vi "FPGA_8a_2ws_BIdireccional_sinWheelsensor.vi"() -> ()   [LabVIEW 2015]
uses:
  <vilib>/LabVIEW Targets/FPGA/cRIO/shared/nicrio_ModuleControls/nicrio_cRIO-9234_DataRatesRing2.ctl
  <vilib>/LabVIEW Targets/FPGA/cRIO/shared/nicrio_ModuleControls/nicrio_BasicConversionTime.ctl
  <vilib>/rvi/Emulation/niFpgaGetClockAttributes.vi
  <vilib>/rvi/Emulation/niFpgaSctlEmulationGetInTimedLoop.vi
  <vilib>/rvi/Emulation/niFpgaEmulationReportErrorSimple.vi
  <vilib>/rvi/Emulation/niFpgaProcessEmulError.vi
  <vilib>/rvi/eio/common/nirviEmuTemplateMethod_errors.vi
  <vilib>/rvi/Emulation/niFpgaCriticalErrorInLSC.vi
  <vilib>/rvi/eio/common/nirviEmuTemplatePropertySet_errors.vi
  <vilib>/rvi/interface/RandomDataEmulation/niFpgaRandomDataHandleErrors.vi
  <vilib>/eio/EIONode/EIONode.xnode
  <vilib>/eio/EIOPropertyNode/EIOPropertyNode.xnode
  <vilib>/rvi/DataTransferAndStorage/Container/XNode/niFpgaContainer.xnode
  <vilib>/rvi/interface/RandomDataEmulation/nirviRandomDataFpgaReadWriteTemplate.vi
  <vilib>/rvi/eio/common/nirviEmuTemplatePropertyGet_errors.vi
  <vilib>/rvi/eio/common/nirviEmuTemplatePropertyGet_noerrors.vi
  <vilib>/rvi/eio/common/nirviEmuTemplatePropertySet_noerrors.vi
panel:
  out "RuedaDetectada2?":bool
  out "RuedaDetectada1?":bool
  out "Numeric 2":i32
  out "WhlCnt1":fxp<+/-,24,-4> format="%.27g"
  in  "Offset_WS1":fxp<+/-,24,-4>=0.000999998301267624 format="%.27g"
  out "Rueda1?":i16
  out "WhlCnt2":fxp<+/-,24,-4> format="%.27g"
  out "Rueda2?":i16
  out "Parar":bool
  out "Nº Ruedas 1":i32
  out "NºRuedas 2":i32
  in  "Offset_WS2":fxp<+/-,24,-4>=0.000999998301267624 format="%.27g"
  in  "Cycles to Filter":u16=5
  in  "Canal cero WS1?":bool=TRUE
  in  "Canal cero WS2?":bool=TRUE
  in  "Conversion Time":T1
  in  "Count(mSec)":u32=2
  in  "Stop":bool
  out "Buffer Underflow":bool
  in  "Digital?":bool=TRUE
  out "medidas":fxp<+/-,24,4>[](array[numeric])
  out "Buffer Overflow":bool
  out "Error Out":errorcluster
  in  "Data Rate":T2=2 items=["51.200 kS/s (NI 9234)"=1, "25.600 kS/s (NI 9234)"=2, "17.067 kS/s (NI 9234)"=3, "12.800 kS/s (NI 9234)"=4, "10.240 kS/s (NI 9234)"=5, "8.533 kS/s (NI 9234)"=6, "7.314 kS/s (NI 9234)"=7, "6.400 kS/s (NI 9234)"=8, "5.689 kS/s (NI 9234)"=9, "5.120 kS/s (NI 9234)"=10, "4.654 kS/s (NI 9234)"=11, "4.267 kS/s (NI 9234)"=12, "3.938 kS/s (NI 9234)"=13, "3.657 kS/s (NI 9234)"=14, "3.413 kS/s (NI 9234)"=15, "3.200 kS/s (NI 9234)"=16, "3.012 kS/s (NI 9234)"=17, "2.845 kS/s (NI 9234)"=18, "2.695 kS/s (NI 9234)"=19, "2.560 kS/s (NI 9234)"=20, "2.438 kS/s (NI 9234)"=21, "2.328 kS/s (NI 9234)"=22, "2.226 kS/s (NI 9234)"=23, "2.133 kS/s (NI 9234)"=24, "2.048 kS/s (NI 9234)"=25, "1.969 kS/s (NI 9234)"=26, "1.896 kS/s (NI 9234)"=27, "1.829 kS/s (NI 9234)"=28, "1.765 kS/s (NI 9234)"=29, "1.707 kS/s (NI 9234)"=30, "1.652 kS/s (NI 9234)"=31]
  out "DC OK":bool
  in  "Fotocélula":bool
  out "Detector de\npresencia":bool
  out "Chassis Temperature":i16
  out "Direccion 0?":bool
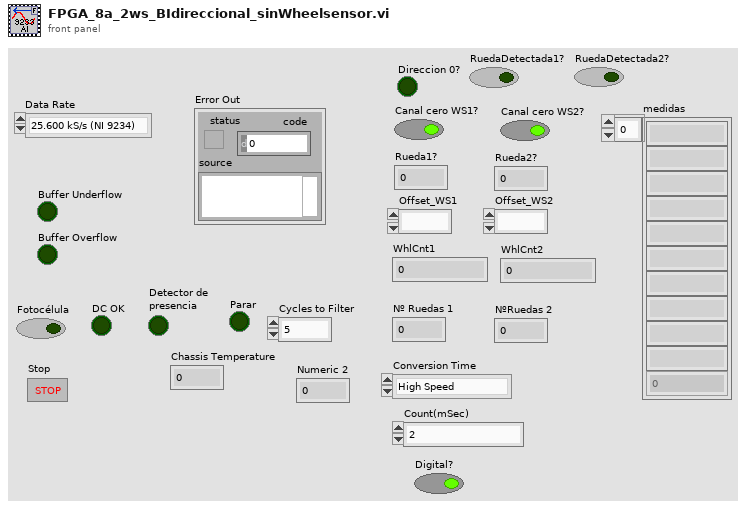
[diagram p1: front panel]
types:
  T1 = typedef "nicrio_BasicConversionTime.ctl" = enum8{"High Speed", "High Resolution"}
  T2 = typedef "nicrio_cRIO-9234_DataRatesRing2.ctl" = u8
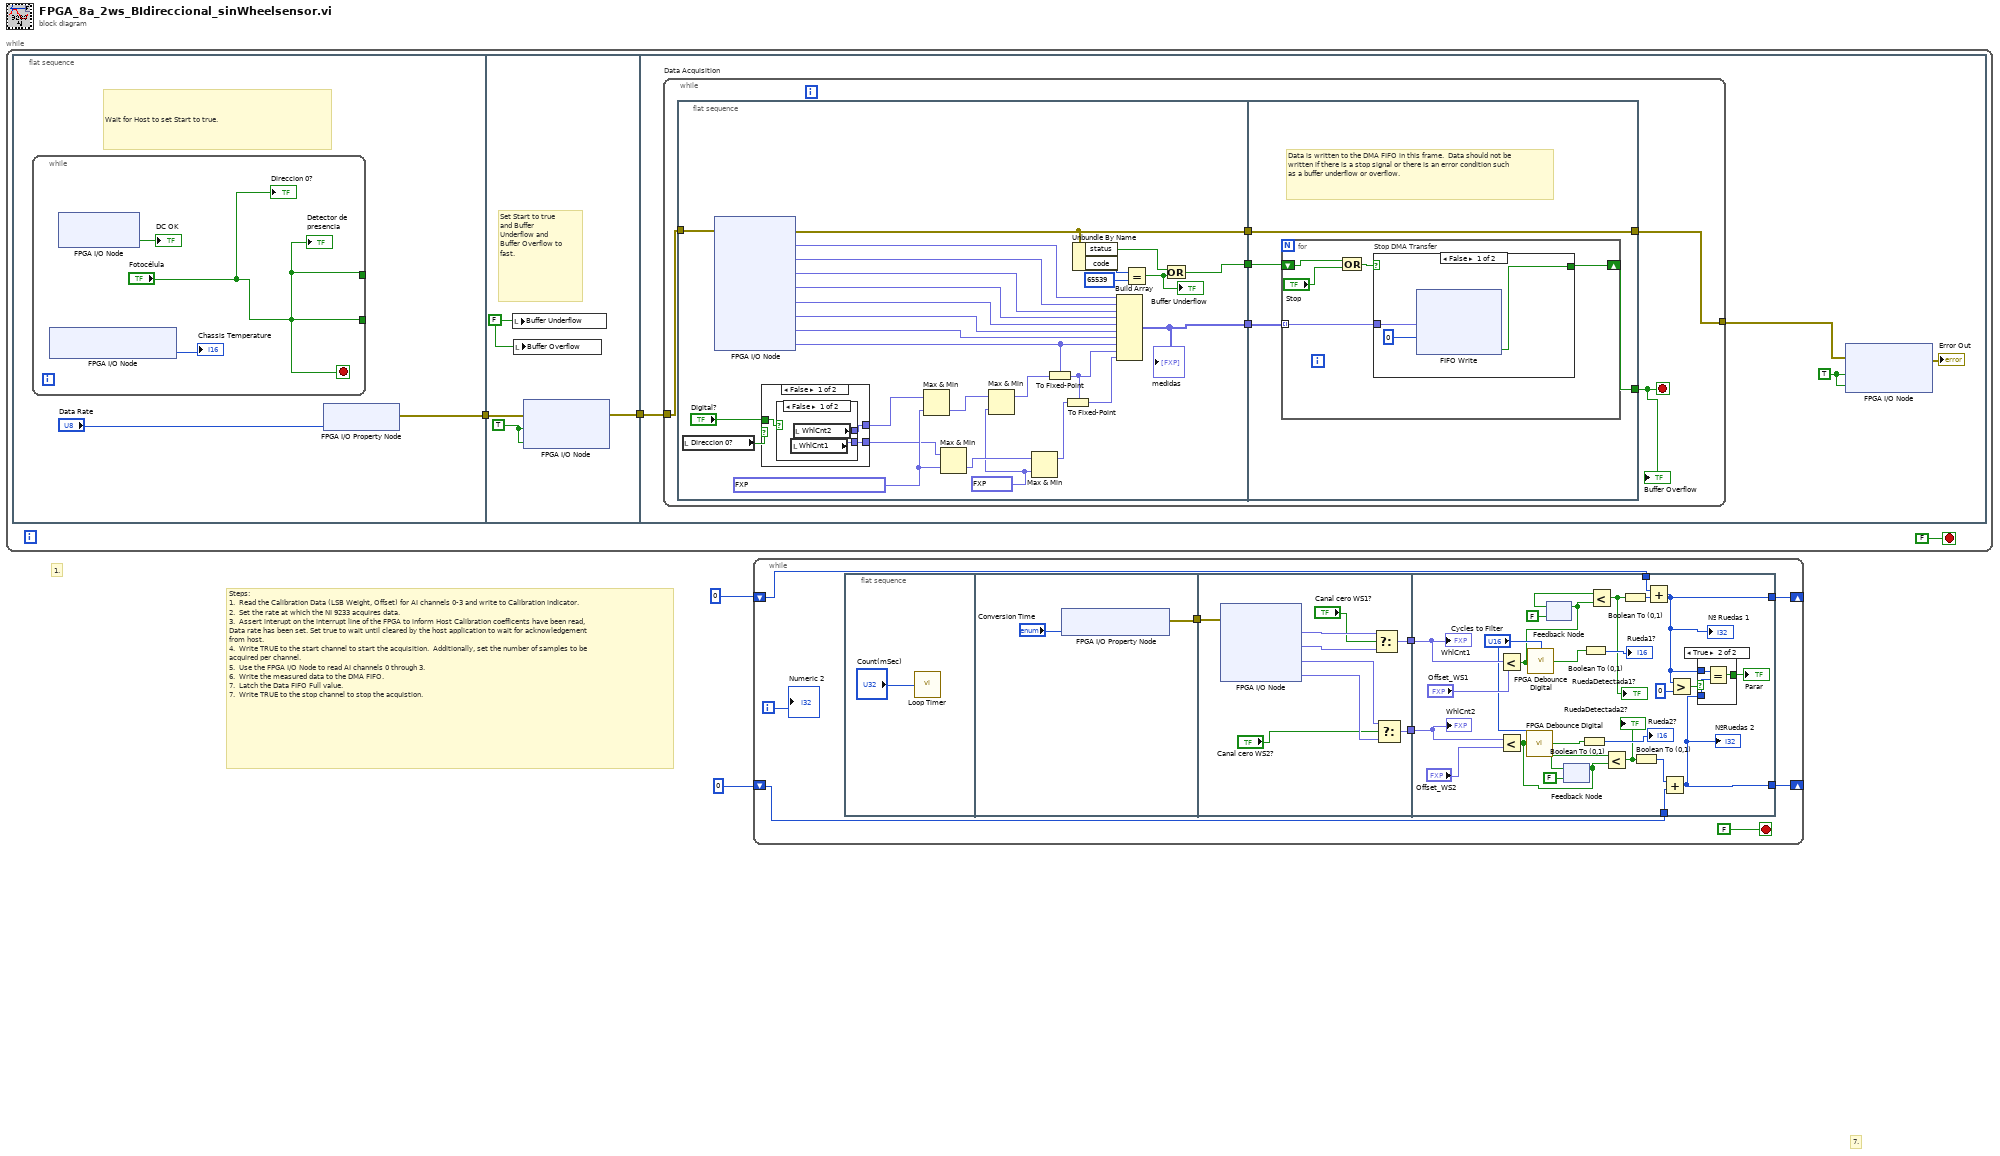
[diagram p0: block diagram]
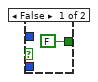
[diagram p2: hidden frame]
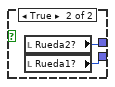
[diagram p3: hidden frame]
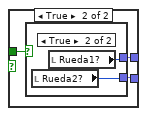
[diagram p4: hidden frame]
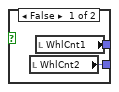
[diagram p5: hidden frame]
diagram:
  # "Steps: \n1.  Read the Calibration Data (LSB Weight, Offset) for AI channels 0-3 and write to Calibration indicator.\n2.  Set the rate at which the NI 9233 acquires data. \n3.  Assert interupt on the interrupt line of the FPGA to inform Host Calibration coefficents have been read, Data rate has been set. Set true to wait until cleared by the host application to wait for acknowledgement from host.\n4.  Write TRUE to the start channel to start the acquisition.  Additionally, set the number of samples to be acquired per channel.\n5.  Use the FPGA I/O Node to read AI channels 0 through 3. \n6.  Write the measured data to the DMA FIFO.\n7.  Latch the Data FIFO Full value.\n7.  Write TRUE to the stop channel to stop the acquistion."
  # "1."
  # "7."
  n1 = while {
    stop <- FALSE stop-if-true
    n2 = flat-sequence "MainSeq" {
      tunnel: [w7] -> w4
      tunnel: w4 -> [w13]
      tunnel: [w12] -> w3
      tunnel: w3 -> [w18]
      frame #0 {
        # "Wait for Host to set Start to true."
        n3 = while "initWait" {
          tunnel: ["Fotocélula"] -> _
          tunnel: ["Fotocélula"] -> _
          stop <- "Fotocélula" stop-if-true
          n4 = xnode "FPGA I/O Node"() -> ("Chassis Temperature"=→"Chassis Temperature":i16)  [unwired: 1 in, 1 out]
          n5 = xnode "FPGA I/O Node"() -> ("Mod3/DI2"=→"DC OK":bool)  [unwired: 2 in, 2 out]
          "Detector de\npresencia" <- "Fotocélula"
          "Direccion 0?" <- "Fotocélula"
        }
        n6 = xnode "FPGA I/O Property Node"("Data Rate"="Data Rate") -> ("error out"=w7:errorcluster)  [unwired: 2 in, 1 out]
      }
      frame #1 {
        w11 = TRUE
        w14 = FALSE ("Late? (Latched)")
        # "Set Start to true and Buffer Underflow and Buffer Overflow to fast."
        n7 = local write "Buffer Underflow"(w14) -> ()
        n8 = local write "Buffer Overflow"(w14) -> ()
        n9 = xnode "FPGA I/O Node"("error in"=w13, "Mod1/Start"=w11, "Mod2/Start"=w11) -> ("error out"=w12:errorcluster)  [unwired: 2 in, 2 out]
      }
      frame #2 {
        w15 = TRUE
        n10 = while "Data Acquisition" {
          tunnel: w18 -> [w22]
          tunnel: [w21] -> w16
          stop <- w19 stop-if-true
          n11 = flat-sequence "Data Acquisition Sequence" {
            tunnel: [w52] -> w24
            tunnel: [w46] -> w23
            tunnel: w22 -> [w51]
            tunnel: [w50] -> w20
            tunnel: w24 -> [w70]
            tunnel: w23 -> [w69]
            tunnel: [w68] -> w19
            tunnel: [w67] -> w21
            tunnel: w20 -> [w67]
            frame #0 {
              w29 = fxp<+/-,44,16> -0.03125 ("y")
              w31 = fxp<+/-,44,16> 0.0312499962747097 ("y")
              n12 = local read "Direccion 0?"() -> (w43:bool)
              n13 = xnode "FPGA I/O Node"("error in"=w51) -> ("error out"=w50:errorcluster, "Mod1/AI0"=w40:fxp<+/-,24,4>, "Mod1/AI1"=w39:fxp<+/-,24,4>, "Mod1/AI2"=w38:fxp<+/-,24,4>, "Mod1/AI3"=w37:fxp<+/-,24,4>, "Mod2/AI0"=w36:fxp<+/-,24,4>, "Mod2/AI1"=w35:fxp<+/-,24,4>, "Mod2/AI2"=w34:fxp<+/-,24,4>, "Mod2/AI3"=w33:fxp<+/-,24,4>)  [unwired: 8 in, 8 out]
              n14 = case shown="False" w43 {
                tunnel: "Digital?" -> [w55 w62]
                tunnel: [w54 w61] -> w27
                tunnel: [w53 w60] -> w26
                frame False {
                  n15 = case shown="False" w55 {
                    tunnel: [w57 w59] -> w54
                    tunnel: [w56 w58] -> w53
                    frame False {
                      n16 = local read "WhlCnt1"() -> (w56:fxp<+/-,24,-4>)
                      n17 = local read "WhlCnt2"() -> (w57:fxp<+/-,24,-4>)
                    }
                    frame True {
                      n18 = local read "Rueda2?"() -> (w59:i16)
                      n19 = local read "Rueda1?"() -> (w58:i16)
                    }
                  }
                }
                frame True {
                  n20 = case shown="True" w62 {
                    tunnel: [w64 w66] -> w61
                    tunnel: [w63 w65] -> w60
                    frame False {
                      n21 = local read "WhlCnt2"() -> (w63:fxp<+/-,24,-4>)
                      n22 = local read "WhlCnt1"() -> (w64:fxp<+/-,24,-4>)
                    }
                    frame True {
                      n23 = local read "Rueda2?"() -> (w65:i16)
                      n24 = local read "Rueda1?"() -> (w66:i16)
                    }
                  }
                }
              }
              n25 = Max & Min(x=w27, y=w31) -> (min(x,y)=w30:fxp<+/-,44,16>)  [unwired: 1 out]
              n26 = Max & Min(x=w26, y=w31) -> (min(x,y)=w32:fxp<+/-,44,16>)  [unwired: 1 out]
              n27 = Max & Min(x=w30, y=w29) -> (max(x,y)=w28:fxp<+/-,44,16>)  [unwired: 1 out]
              n28 = Max & Min(x=w32, y=w29) -> (max(x,y)=w25:fxp<+/-,44,16>)  [unwired: 1 out]
              n29 = To Fixed-Point(fixed-point type=w33, number=w28) -> (fixed-point=w42:fxp<+/-,24,4>)
              n30 = To Fixed-Point(fixed-point type=w42, number=w25) -> (fixed-point=w41:fxp<+/-,24,4>)
              n31 = Unbundle By Name(w50) -> ("status"=w45:bool, "code"=w49:i32)
              n32 = Build Array(w40, w39, w38, w37, w36, w35, w34, w33, w42, w41) -> (w52:fxp<+/-,24,4>[])
              "medidas" <- w52
              n33 = Equal?(x=w49, y=65539) -> (x = y?=w47:bool)
              "Buffer Underflow" <- w47
              n34 = Or(x=w45, y=w47) -> (x .or. y?=w46:bool)
            }
            frame #1 {
              # "Data is written to the DMA FIFO in this frame.  Data should not be written if there is a stop signal or there is an error condition such as a buffer underflow or overflow."
              n35 = for "DMAWriteLoop" {
                tunnel: w70 -> [w75] mode=indexing
                shift-right: [w74] -> w68
                shift-left: w69 -> [w73]
                n36 = Compound Arithmetic op=OR(w73, "Stop") -> (w72:bool)
                n37 = case "Stop DMA Transfer" shown="False" w72 {
                  selector: w72 -> [_ w79]
                  tunnel: w75 -> [w76 _]
                  tunnel: [w78 w79] -> w74
                  frame False {
                    n38 = xnode ("FIFO Write")("Element"=w76, "Timeout"=0) -> ("Timed Out?"=w78:bool)  [unwired: 1 in, 1 out]
                  }
                  frame True {
                  }
                }
              }
            }
          }
          "Buffer Overflow" <- w19
        }
        n39 = xnode "FPGA I/O Node"("error in"=w16, "Mod1/Stop"=w15, "Mod2/Stop"=w15) -> ("error out"=→"Error Out":errorcluster)  [unwired: 2 in, 2 out]
      }
    }
  }
  n40 = while {
    shift-right: [w85] -> _
    shift-left: 0 -> [w84]
    shift-right: [w82] -> _
    shift-left: 0 -> [w83]
    i -> [w81]
    stop <- FALSE stop-if-true
    n41 = flat-sequence {
      tunnel: [w90] -> w87
      tunnel: [w100] -> w88
      tunnel: w87 -> [w94]
      tunnel: [w97] -> w86
      tunnel: w88 -> [w126]
      tunnel: w86 -> [w124]
      tunnel: [w114] -> w85
      tunnel: w84 -> [w121]
      tunnel: w83 -> [w119]
      tunnel: [w113] -> w82
      frame #0 {
        n42 = call "Loop Timer"("Count(mSec)"="Count(mSec)") -> ()  [unwired: 1 out]
      }
      frame #1 {
        n43 = xnode "FPGA I/O Property Node"("Conversion Time"="Conversion Time") -> ("error out"=w90:errorcluster)  [unwired: 2 in, 1 out]
      }
      frame #2 {
        n44 = xnode "FPGA I/O Node"("error in"=w94) -> ("Mod4/AI0"=w99:fxp<+/-,24,-4>, "Mod4/AI1"=w98:fxp<+/-,24,-4>, "Mod4/AI2"=w96:fxp<+/-,24,-4>, "Mod4/AI3"=w95:fxp<+/-,24,-4>)  [unwired: 4 in, 5 out]
        n45 = Select(t=w99, s="Canal cero WS1?", f=w98) -> (s? t:f=w100:fxp<+/-,24,-4>)
        n46 = Select(t=w96, s="Canal cero WS2?", f=w95) -> (s? t:f=w97:fxp<+/-,24,-4>)
      }
      frame #3 {
        n47 = Less?(x=w126, y="Offset_WS1") -> (x < y?=w106:bool)
        n48 = Less?(x=w124, y="Offset_WS2") -> (x < y?=w104:bool)
        n49 = call "FPGA Debounce Digital.vi"("Input Signal"=w104, "Cycles to Filter"="Cycles to Filter") -> ("Output Filtered Signal"=w103:bool)
        n50 = call "FPGA Debounce Digital.vi"("Input Signal"=w106, "Cycles to Filter"="Cycles to Filter") -> ("Output Filtered Signal"=w105:bool)
        n51 = feedback-in #1(w106) -> ()
        n52 = feedback #1(FALSE) -> (w122:bool)
        n53 = feedback #2(FALSE) -> (w115:bool)
        n54 = feedback-in #2(w104) -> ()
        n55 = Boolean To (0,1)(Boolean=w103) -> (0, 1=→"Rueda2?":i16)
        n56 = Boolean To (0,1)(Boolean=w105) -> (0, 1=→"Rueda1?":i16)
        n57 = Less?(x=w122, y=w106) -> (x < y?=w102:bool)
        "RuedaDetectada1?" <- w102
        n58 = Less?(x=w115, y=w104) -> (x < y?=w101:bool)
        "RuedaDetectada2?" <- w101
        n59 = Boolean To (0,1)(Boolean=w102) -> (0, 1=w108:i16)
        n60 = Boolean To (0,1)(Boolean=w101) -> (0, 1=w111:i16)
        n61 = Add(x=w121, y=w108) -> (x+y=w114:i32)
        "Nº Ruedas 1" <- w114
        n62 = Add(x=w111, y=w119) -> (x+y=w113:i32)
        "NºRuedas 2" <- w113
        n63 = Greater?(x=w114, y=i64 0) -> (0:w116:bool)
        n64 = case shown="True" w116 {
          tunnel: w113 -> [_ w130]
          tunnel: w114 -> [_ w129]
          tunnel: [FALSE w128] -> w118
          frame False {
          }
          frame True {
            n65 = Equal?(x=w129, y=w130) -> (x = y?=w128:bool)
          }
        }
        "Parar" <- w118
        "WhlCnt1" <- w126
        "WhlCnt2" <- w124
      }
    }
    "Numeric 2" <- w81
  }
